vi "test_shared_var.vi"() -> ()   [LabVIEW 2018]
panel:
  in  "setpos":i16
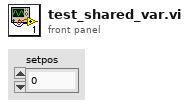
[diagram p1: front panel]
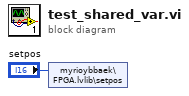
[diagram p0: block diagram]
diagram:
  n1 = shared-variable "myrioybbaek\\FPGA.lvlib\\setpos"("setpos") -> ()  [unwired: 1 in, 1 out]
